vi "CAN Get Comm State.vi"(8 "error in (no error)":errorcluster, 11 "CAN Refs and Settings":T1[](array[typedef])) -> (0 "error out":errorcluster, 3 "CAN Refs and Settings out":T1[](array[typedef]))   [LabVIEW 2018, in "NI-XNET Monitor Engine.lvlib"]
uses:
  NI-XNET Monitor Engine.lvlib
  typedefs/CANBus.Settings.ctl
  Bus Load/CANBus/CANBus_Load_Calculator.lvclass
  <vilib>/NI/NIVS Inline Async API/_Data Access Engine/Data Access Engine/Types/Write.DVR.ctl
  <vilib>/NI/NIVS Inline Async API/_Data Access Engine/Access Type Classes/Write/Write.lvclass
  <vilib>/NI/NIVS Inline Async API/_Data Access Engine/Access Type Classes/Write/Write.lvclass/Write.ctl
  <vilib>/NI/NIVS Inline Async API/_Data Access Engine/Data Access Engine/Methods/Write.Data.vi
  <vilib>/NI/NIVS Inline Async API/_Data Access Engine/Access Type Classes/Write/Write.ProcessData.vi
  <vilib>/xnet/xnet.llb/XNET Read (Frame CAN).vi
  <vilib>/xnet/xnet.llb/XNET Read (State CAN Comm).vi
  <vilib>/NI/NIVS Inline Async API/_Data Access Engine/Data Access Engine/Data Access Engine.lvclass
  Bus Load/XNET-Bus-Load-Calculator.lvlib
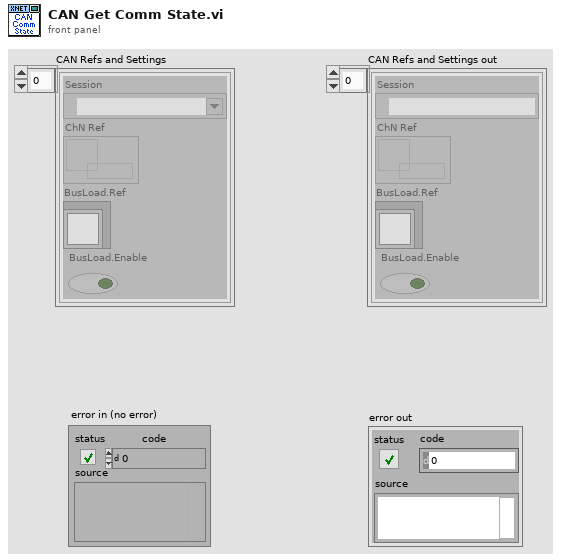
[diagram p1: front panel]
types:
  T1 = typedef "NI-XNET Monitor Engine.lvlib/CANBus.Settings.ctl" = cluster{"Session":refnum<k21>, "ChN Ref":T2, "BusLoad.Ref":refnum<class "CANBus_Load_Calculator.lvclass">, "BusLoad.Enable":bool}
  T2 = typedef "Data Access Engine.lvlib/Data Access Engine.lvclass/Write.DVR.ctl" = refnum<data-value>
  T3 = typedef "XNET Frame CAN.ctl" = cluster{"timestamp":timestamp, "payload":u8[], "identifier":u32, "type":T4, "extended?":bool, "echo?":bool}
  T4 = typedef "XNET Frame Type CAN.ctl" = u8
  T5 = typedef "XNET CAN Comm.ctl" = cluster{"fault code":i32, "fault?":bool, "communication state":T6, "last error":T7, "receive error counter":u8, "transmit error counter":u8, "transceiver error?":bool, "sleep?":bool}
  T6 = typedef "XNET CAN Comm State.ctl" = u8
  T7 = typedef "XNET CAN Last Err.ctl" = u8
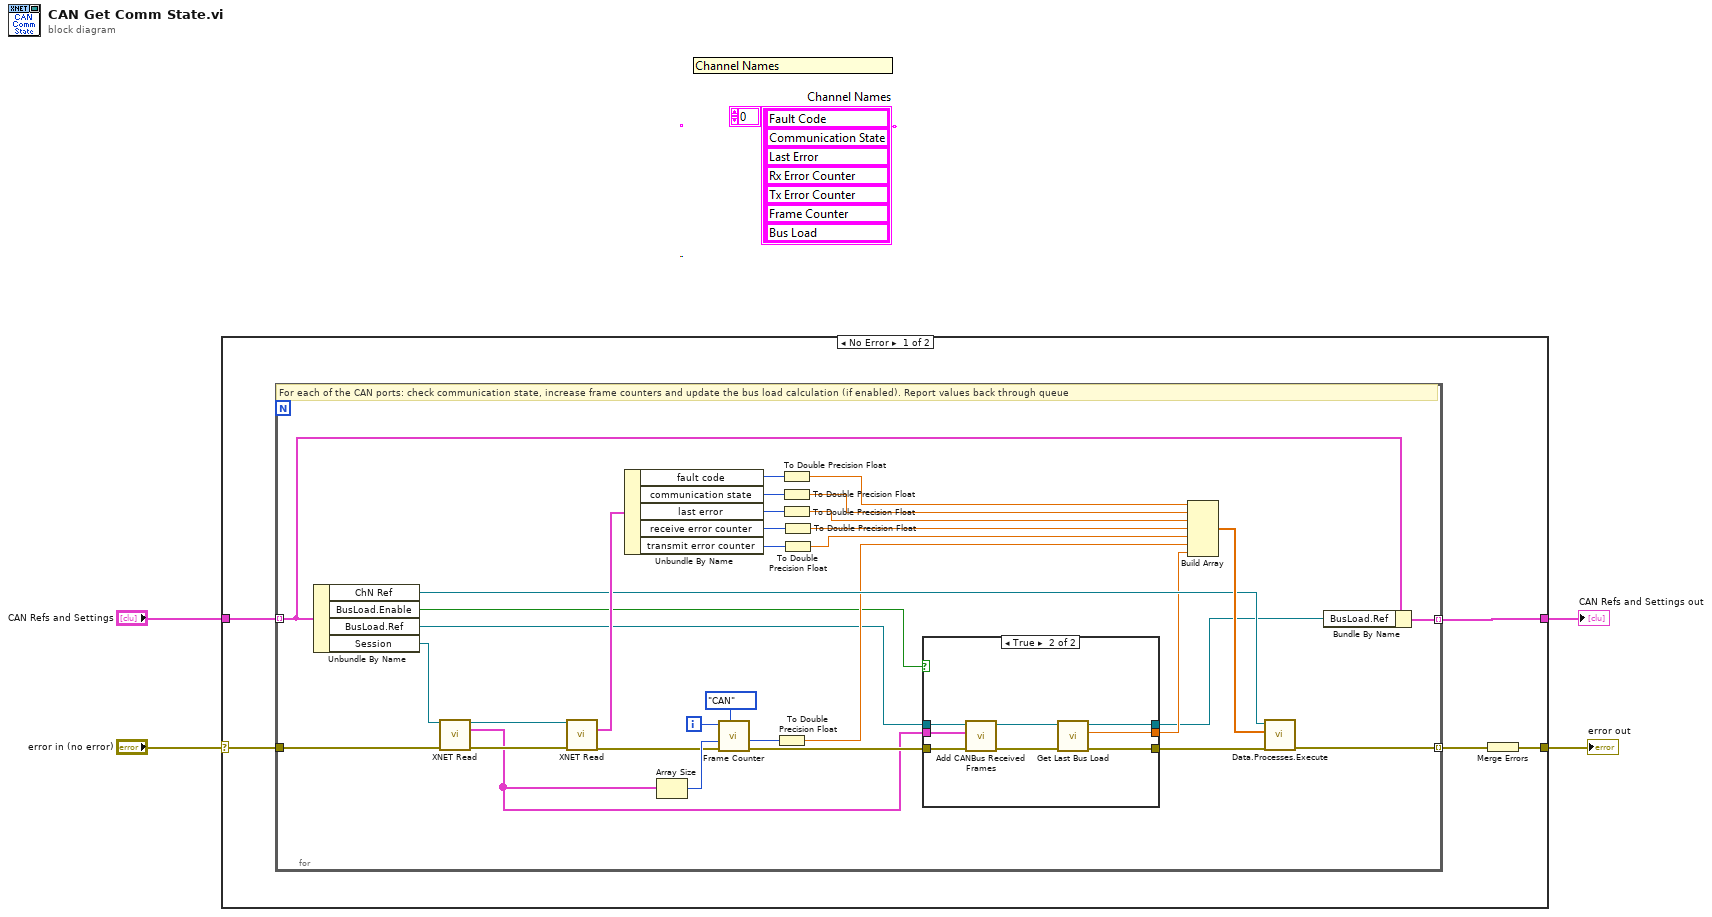
[diagram p0: block diagram]
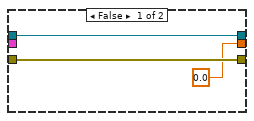
[diagram p2: hidden frame]
diagram:
  n1 = case shown="No Error" "error in (no error)" {
    selector: "error in (no error)" -> [w6 w55]
    tunnel: "CAN Refs and Settings" -> [w9 w54]
    tunnel: [w7 w55] -> w3
    tunnel: [w5 w54] -> w1
    frame No Error {
      n2 = for {
        tunnel: w9 -> [w12] mode=indexing
        tunnel: [w42] -> w8 mode=indexing
        tunnel: w6 -> [w16]
        tunnel: [w10] -> w5 mode=indexing
        i -> [w38]
        # "For each of the CAN ports: check communication state, increase frame counters and update the bus load calculation (if enabled). Report values back through queue"
        n3 = Unbundle By Name(w12) -> ("ChN Ref"=w22:T2, "BusLoad.Enable"=w17:bool, "BusLoad.Ref"=w15:refnum<class "CANBus_Load_Calculator.lvclass">, "Session"=w36:refnum<k21>)
        n4 = call-poly <vilib>:"XNET Read.vi"("session in"=w36, "error in (no error)"=w16) -> ("session out"=w40:refnum<k21>, "data"=w13:T3[], "error out"=w24:errorcluster)  [unwired: 10 in, 1 out]
        n5 = call-poly <vilib>:"XNET Read.vi"("session in"=w40, "error in (no error)"=w24) -> ("CAN comm"=w35:T5, "error out"=w23:errorcluster)  [unwired: 11 in, 1 out]
        n6 = Unbundle By Name(w35) -> ("fault code"=w34:i32, "communication state"=w33:T6, "last error"=w32:T7, "receive error counter"=w31:u8, "transmit error counter"=w30:u8)
        n7 = Array Size(array=w13) -> (size(s)=w39:i32)
        n8 = call "Frame Counter.vi"("bus type"=enum16{"CAN", "FlexRay", "LIN"}."CAN", "error in (no error)"=w23, "new frames"=w39, "bus index (bus count for init)"=w38) -> ("error out"=w21:errorcluster, "total frames"=w20:u32)  [unwired: 6 in]
        n9 = To Double Precision Float(number=w20) -> (double precision float=w19:dbl)
        n10 = To Double Precision Float(number=w34) -> (double precision float=w29:dbl)
        n11 = To Double Precision Float(number=w33) -> (double precision float=w28:dbl)
        n12 = To Double Precision Float(number=w32) -> (double precision float=w27:dbl)
        n13 = To Double Precision Float(number=w31) -> (double precision float=w26:dbl)
        n14 = To Double Precision Float(number=w30) -> (double precision float=w25:dbl)
        n15 = case shown="True" w17 {
          tunnel: w21 -> [w45 w51]
          tunnel: [w45 w50] -> w18
          tunnel: w15 -> [w43 w49]
          tunnel: [0.0 ("Bus Load (%)") w48] -> w14
          tunnel: w13 -> [_ w47]
          tunnel: [w43 w46] -> w11
          frame False {
          }
          frame True {
            n16 = call "Add CANBus Received Frames.vi"("error in (no error)"=w51, "CAN Frames"=w47, "Load Calculator in"=w49) -> ("error out"=w52:errorcluster, "Load Calculator out"=w53:refnum<class "CANBus_Load_Calculator.lvclass">)  [unwired: 7 in]
            n17 = call "Get Last Bus Load.vi"("error in (no error)"=w52, "Load Calculator in"=w53) -> ("error out"=w50:errorcluster, "Bus Load (%)"=w48:dbl, "Load Calculator out"=w46:refnum<class "CANBus_Load_Calculator.lvclass">)  [unwired: 7 in]
          }
        }
        n18 = Build Array(w29, w28, w27, w26, w25, w19, w14) -> (w41:dbl[])
        n19 = call-poly <vilib>:"Data.Processes.Execute.vi"("error in (no error)"=w18, "Values"=w41, "Ref"=w22) -> ("error out"=w42:errorcluster)  [unwired: 8 in]
        n20 = Bundle By Name(cluster=w12, "BusLoad.Ref"=w11) -> (w10:T1)
      }
      n21 = Merge Errors(w8) -> (w7:errorcluster)
    }
    frame Error {
    }
  }
  "error out" <- w3
  "CAN Refs and Settings out" <- w1
